vi "Load Limits File.vi"(8 "error in (no error)":errorcluster, 11 "Test Number and Bin Generator In":refnum<class "Test Number and Bin Generator.lvclass">=refnum) -> (0 "error out":errorcluster, 3 "Test Number and Bin Generator Out":refnum<class "Test Number and Bin Generator.lvclass">)   [LabVIEW 2018, in "Test Number and Bin Generator.lvlib" / "Test Number and Bin Generator.lvclass"]
uses:
  Test Number and Bin Generator.lvclass
  Test Number and Bin Generator.lvclass/Test Number and Bin Generator.ctl
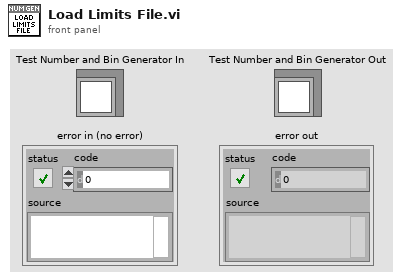
[diagram p1: front panel]
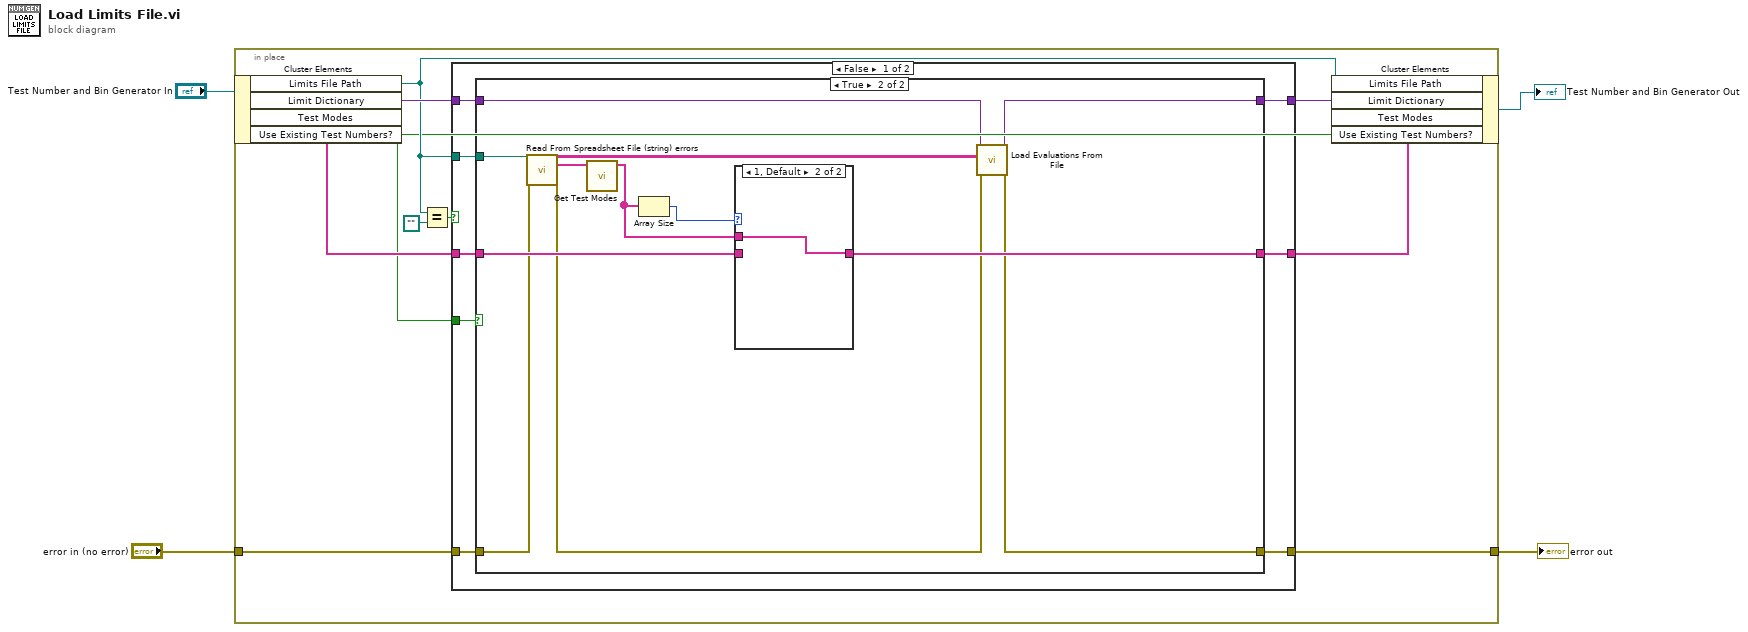
[diagram p0: block diagram]
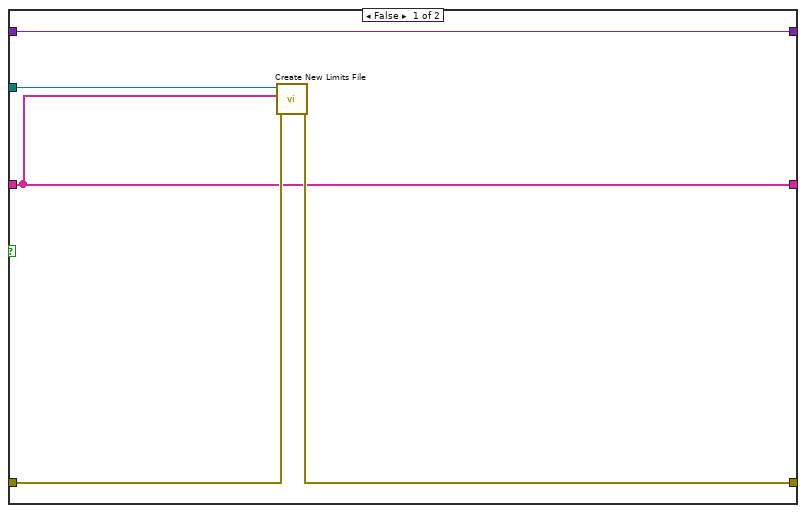
[diagram p2: hidden frame]
diagram:
  n1 = in-place {
    in-place-border: "error in (no error)" -> [w7]
    in-place-border: [w6] -> w1
    n2 = in-place-cluster #1("Test Number and Bin Generator In") -> ("Limits File Path"=w12:path, "Limit Dictionary"=w14:variant, "Test Modes"=w10:string[], "Use Existing Test Numbers?"=w5:bool)
    n3 = Equal?(x=w12, y=path "") -> (x = y?=w11:bool)
    n4 = case shown="False" w11 {
      tunnel: w14 -> [w22 w44]
      tunnel: [w21 w44] -> w13
      tunnel: w12 -> [w20 _]
      tunnel: w10 -> [w19 w43]
      tunnel: [w18 w43] -> w9
      tunnel: w7 -> [w17 w42]
      tunnel: [w16 w42] -> w6
      tunnel: w5 -> [w15 _]
      frame False {
        n5 = case shown="True" w15 {
          tunnel: w22 -> [w27 w38]
          tunnel: [w27 w37] -> w21
          tunnel: w20 -> [w26 w36]
          tunnel: w19 -> [w23 w33]
          tunnel: [w23 w32] -> w18
          tunnel: w17 -> [w25 w31]
          tunnel: [w24 w29] -> w16
          frame False {
            n6 = call "Create New Limits File.vi"("error in (no error)"=w25, "Test Modes"=w23, "Limits File Path"=w26) -> ("error out"=w24:errorcluster)  [unwired: 8 in]
          }
          frame True {
            n7 = call "Read From Spreadsheet File (string) errors.vi"("file path (dialog if empty)"=w36, "error in (not an error)"=w31) -> ("all rows"=w39:string[][], "first row"=w35:string[], "error out"=w30:errorcluster)  [unwired: 20 in, 3 out]
            n8 = call "Get Test Modes.vi"("First Row"=w35) -> ("Test Modes Out"=w28:string[])  [unwired: 10 in]
            n9 = Array Size(array=w28) -> (size(s)=w34:i32)
            n10 = case shown="1, Default" w34 {
              tunnel: w33 -> [w40 _]
              tunnel: [w40 w41] -> w32
              tunnel: w28 -> [_ w41]
              frame 0 {
              }
              frame 1, Default {
              }
            }
            n11 = call "Load Evaluations From File.vi"("error in (no error)"=w30, "all rows"=w39, "Limit Dictionary in"=w38) -> ("error out"=w29:errorcluster, "Limit Dictionary out"=w37:variant)  [unwired: 7 in]
          }
        }
      }
      frame True {
      }
    }
    n12 = in-place-cluster #1("Limits File Path"=w12, "Limit Dictionary"=w13, "Test Modes"=w9, "Use Existing Test Numbers?"=w5) -> (→"Test Number and Bin Generator Out":refnum<class "Test Number and Bin Generator.lvclass">)
  }
  "error out" <- w1
